vi "log_analysis_cpu-mem.vi"() -> ()   [LabVIEW 2019]
panel:
  out "memory Graph 2":dbl[][](graph)
  in  "y":bool
  in  "file path (use dialog)":path=path "C:/AGV/Log/2021/Log_20210216-1751.txt"
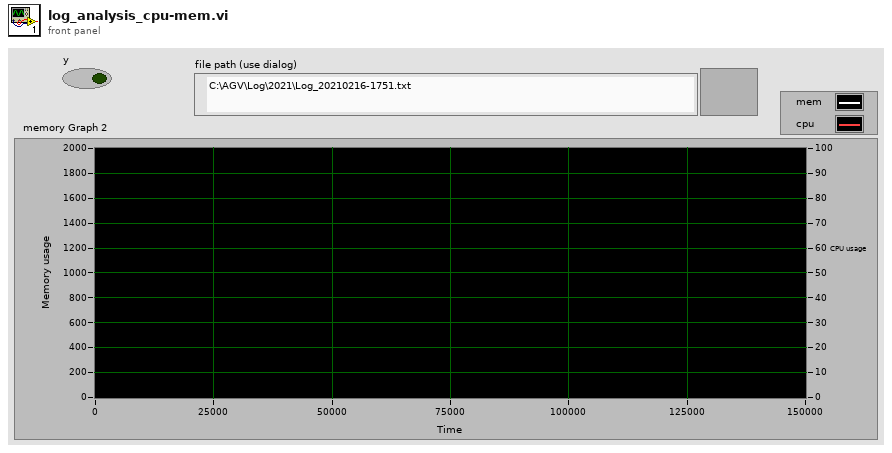
[diagram p1: front panel]
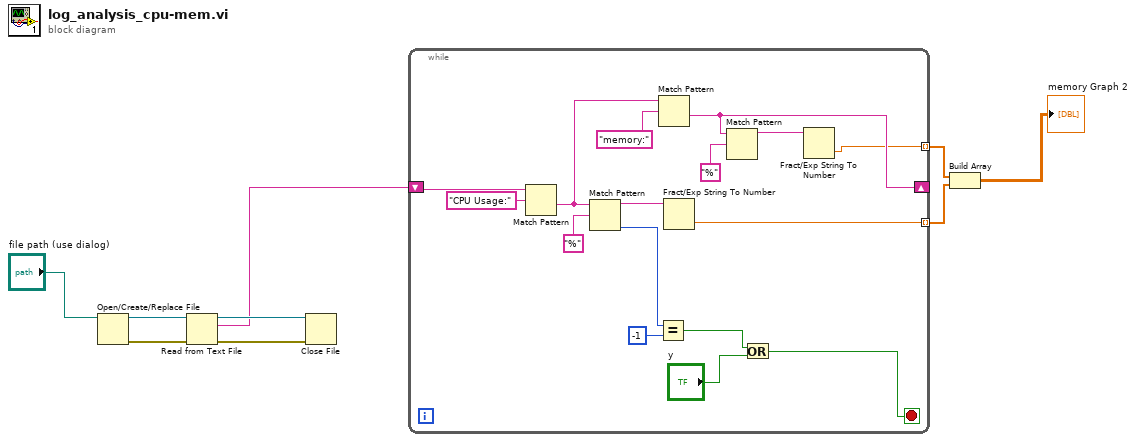
[diagram p0: block diagram]
diagram:
  n1 = Open/Create/Replace File(file path (use dialog)="file path (use dialog)") -> (refnum out=w6:refnum<file>, error out=w9:errorcluster)  [unwired: 5 in, 1 out]
  n2 = Read from Text File(file (use dialog)=w6, error in=w9) -> (refnum out=w7:refnum<file>, text=w4:string, error out=w8:errorcluster)  [unwired: 2 in, 1 out]
  n3 = Close File(refnum=w7, error in=w8) -> ()  [unwired: 2 out]
  n4 = while {
    shift-right: [w17] -> _
    shift-left: w4 -> [w25]
    tunnel: [w11] -> w2 mode=indexing
    tunnel: [w10] -> w3 mode=indexing
    stop <- w13 stop-if-true
    n5 = Match Pattern(string=w25, regular expression="CPU Usage:") -> (after substring=w20:string)  [unwired: 1 in, 3 out]
    n6 = Match Pattern(string=w20, regular expression="%") -> (before substring=w22:string, offset past match=w16:i32)  [unwired: 1 in, 2 out]
    n7 = Equal?(x=w16, y=-1) -> (x = y?=w14:bool)
    n8 = Match Pattern(string=w20, regular expression="memory:") -> (after substring=w17:string)  [unwired: 1 in, 3 out]
    n9 = Fract/Exp String To Number(string=w22) -> (number=w11:dbl)  [unwired: 3 in, 1 out]
    n10 = Match Pattern(string=w17, regular expression="%") -> (before substring=w18:string)  [unwired: 1 in, 3 out]
    n11 = Or(x=w14, y="y") -> (x .or. y?=w13:bool)
    n12 = Fract/Exp String To Number(string=w18) -> (number=w10:dbl)  [unwired: 3 in, 1 out]
  }
  n13 = Build Array(w3, w2) -> (→"memory Graph 2":dbl[][])
